vi "GetGyro.vi"() -> (2 "Angular Rate":dbl, 3 "Angle":dbl, 4 "Raw Angle":dbl)   [LabVIEW 2013]
uses:
  Robot Global Data.vi
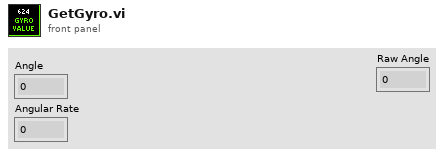
[diagram p1: front panel]
types:
  T1 = typedef "WPI_GyroDevRef.ctl" = cluster{"DevStatus":errorcluster, "Analog Module":T2, "Analog Channel":T3, "Offset":dbl, "Gain (VoltsPerDegree/Second)":dbl}
  T2 = typedef "FPGA_TypedefAnalogModule.ctl" = enum16{"Analog Module 1", "Analog Module 2"}
  T3 = typedef "FPGA_AIChannel.ctl" = enum8{"AI 1", "AI 2", "AI 3", "AI 4", "AI 5", "AI 6", "AI 7", "AI 8", "Invalid"}
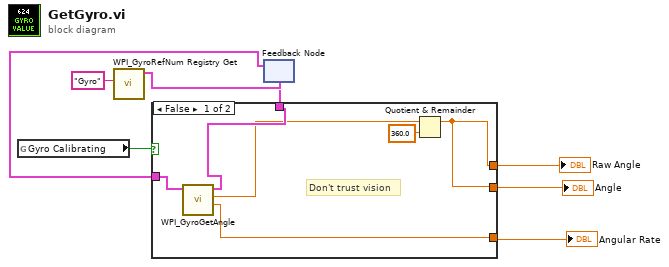
[diagram p0: block diagram]
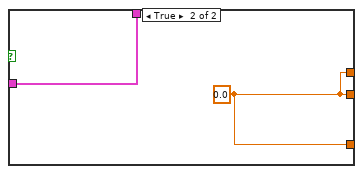
[diagram p2: hidden frame]
diagram:
  n1 = global read "Robot Global Data.vi" "Gyro Calibrating"() -> (w5:bool)
  n2 = call <vilib>:"WPI_GyroRefNum Registry Get.vi"("refnum name"="Gyro") -> ("GyroDevRef"=w4:T1)  [unwired: 9 in, 1 out]
  n3 = feedback #1(w4) -> (w3:T1)
  n4 = case shown="False" w5 {
    tunnel: w3 -> [w13 w16]
    tunnel: [w9 w15] -> w7
    tunnel: [w14 w15] -> w6
    tunnel: [w12 w16] -> w2
    tunnel: [w9 w15] -> w1
    frame False {
      # "Don't trust vision"
      n5 = call <vilib>:"WPI_GyroGetAngle.vi"("GyroDevRef"=w13) -> ("Angular Rate"=w14:dbl, "Angle"=w10:dbl, "GyroDevRef"=w12:T1)  [unwired: 7 in, 1 out]
      n6 = Quotient & Remainder(x=w10, y=360.0) -> (x-y*floor(x/y)=w9:dbl)  [unwired: 1 out]
    }
    frame True {
      w15 = 0.0
    }
  }
  "Angle" <- w7
  "Angular Rate" <- w6
  "Raw Angle" <- w1
  n7 = feedback-in #1(w2) -> ()
